vi "Filter_3Way.vi"(0 "Data IN":i32[](array[numeric]), 1 "DataRate (SPS)":dbl, 5 "Low Pass Filter Settings":T2, 7 "High Pass Filter Settings":T2, 9 "Notch Filter":enum16{"50Hz", "60Hz"}(ring)=enum."60Hz", 11 "Notch Order":i32, 12 "LPF Enable":bool, 13 "50/60 Notch Enable":bool, 14 "HPF Enable":bool) -> (4 "Data OUT":dbl[](array[numeric]))   [LabVIEW 2010]
doc: "This VI provides options for performing digitial filtering on the input data.\nOptions are provided for a single filter for each of the following:\n - Low Pass Filter\n - High Pass Filter\n - Notch Filter for 50/60Hz removal\n\nInputs;\nData IN - (I32[]) data to be filtered\nLPF Enable - (bool) TRUE = turn filter ON\nLow Pass Filter Settings - LPF parameters\nHPF Enable - (bool) TRUE = turn filter ON\nHigh Pass Filter Settings - HPF parameters\n50/60 Notch Enable - (bool) TRUE = turn filter ON\nNotch Filer - (enum) specify which filter to use\nNotch Order - (I32) notch filter order\nDataRate(SPS) - (DBL) data rate of input data\n\nOutput:\nData OUT - (DBL[]) filtered data"
uses:
  TYP_FilterSettings.ctl
  <vilib>/Analysis/3filter.llb/Filter Passband Type.ctl
  <vilib>/Analysis/3filter.llb/Butterworth Filter (DBL).vi
  <vilib>/Analysis/NI_AALBase.lvlib
panel:
  in  "50/60 Hz Notch Limits":T1={"50Hz Cutoff Freq"={"High"=53.0, "Low "=47.0}, "60Hz Cutoff Freq"={"High"=63.0, "Low "=57.0}} {"60Hz Cutoff Freq"."Low" format="%#_gHz"; "60Hz Cutoff Freq"."High" format="%#_gHz"; "50Hz Cutoff Freq"."Low" format="%#_gHz"; "50Hz Cutoff Freq"."High" format="%#_gHz"}
  # "Front Panel Constant (need to set as defaults)"
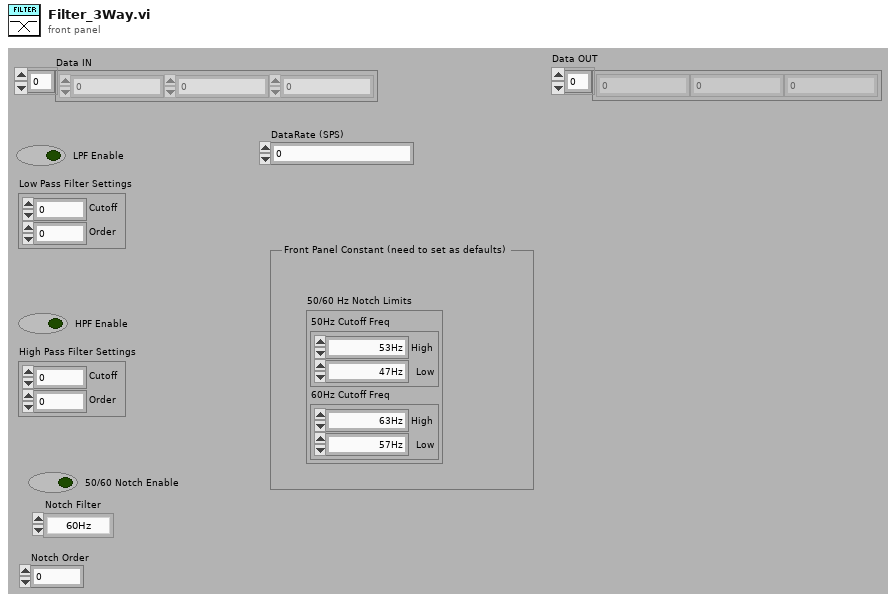
[diagram p1: front panel]
types:
  T1 = cluster{"50Hz Cutoff Freq":cluster{"High":dbl, "Low ":dbl}, "60Hz Cutoff Freq":cluster{"High":dbl, "Low ":dbl}}
  T2 = typedef "TYP_FilterSettings.ctl" = cluster{"Cutoff":dbl, "Order":i32}
  T3 = typedef "NI_AALBase.lvlib/Filter Passband Type.ctl" = enum32{"Lowpass", "Highpass", "Bandpass", "Bandstop"}
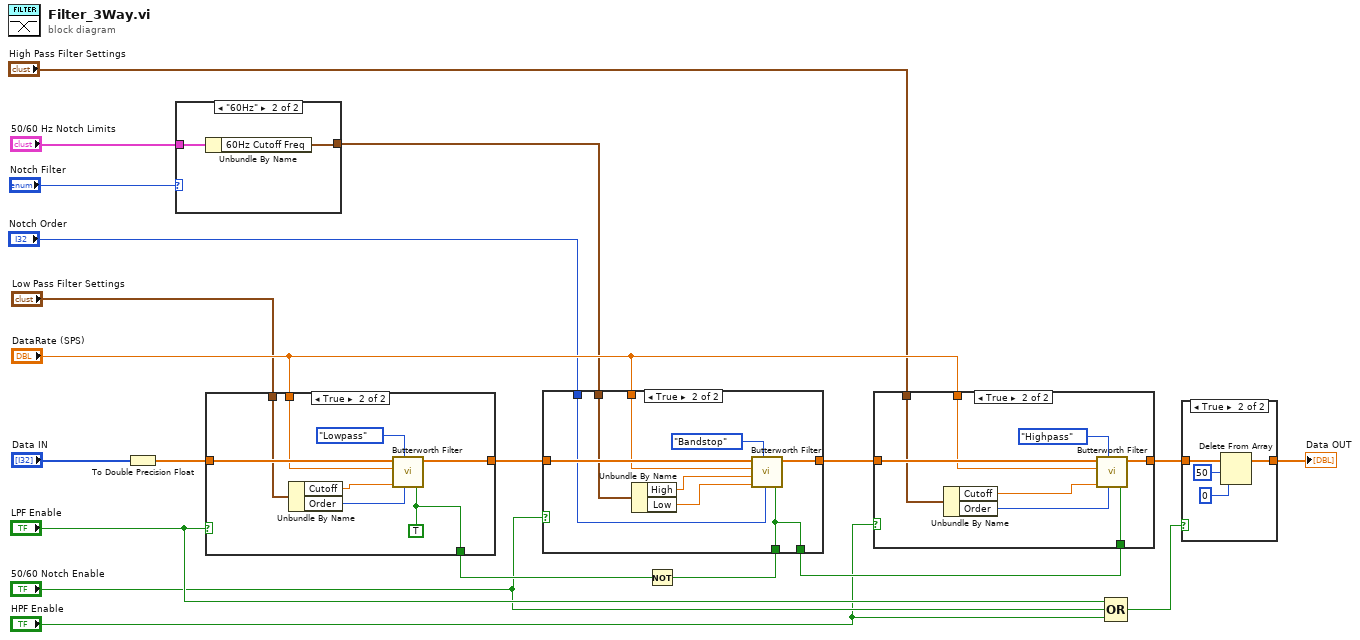
[diagram p0: block diagram]
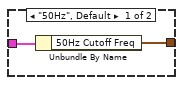
[diagram p3: hidden frame]
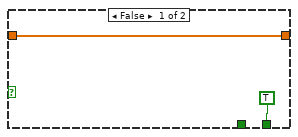
[diagram p5: hidden frame]
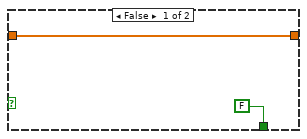
[diagram p6: hidden frame]
diagram:
  n1 = To Double Precision Float(number="Data IN") -> (double precision float=w17:dbl[])
  n2 = case shown="\"60Hz\"" "Notch Filter" {
    tunnel: "50/60 Hz Notch Limits" -> [w22 w24]
    tunnel: [w21 w23] -> w11
    frame "50Hz", Default {
      n3 = Unbundle By Name(w22) -> ("50Hz Cutoff Freq"=w21:cluster{"High":dbl, "Low ":dbl})
    }
    frame "60Hz" {
      n4 = Unbundle By Name(w24) -> ("60Hz Cutoff Freq"=w23:cluster{"High":dbl, "Low ":dbl})
    }
  }
  n5 = case shown="True" "LPF Enable" {
    tunnel: w17 -> [w26 w33]
    tunnel: [w26 w34] -> w19
    tunnel: "DataRate (SPS)" -> [_ w31]
    tunnel: "Low Pass Filter Settings" -> [_ w30]
    tunnel: [FALSE w27] -> w9
    frame False {
    }
    frame True {
      w27 = TRUE ("init/cont (init:F)")
      n6 = Unbundle By Name(w30) -> ("Cutoff"=w29:dbl, "Order"=w28:i32)
      n7 = call-poly <vilib>:"Butterworth Filter.vi"("init/cont (init:F)"=w27, "order"=w28, "filter type"=Filter_Passband_Type."Lowpass", "low cutoff freq: fl"=w29, "sampling freq: fs"=w31, "X"=w33) -> ("Filtered X"=w34:dbl[])  [unwired: 2 in, 1 out]
    }
  }
  n8 = Not(x=w9) -> (.not. x?=w8:bool)
  n9 = case shown="True" "50/60 Notch Enable" {
    tunnel: w19 -> [w36 w44]
    tunnel: [w36 w45] -> w18
    tunnel: "DataRate (SPS)" -> [_ w42]
    tunnel: "Notch Order" -> [_ w41]
    tunnel: w11 -> [_ w40]
    tunnel: w8 -> [_ w37]
    tunnel: [TRUE w37] -> w7
    frame False {
    }
    frame True {
      n10 = Unbundle By Name(w40) -> ("High"=w39:dbl, "Low"=w38:dbl)
      n11 = call-poly <vilib>:"Butterworth Filter.vi"("init/cont (init:F)"=w37, "order"=w41, "filter type"=Filter_Passband_Type."Bandstop", "low cutoff freq: fl"=w38, "high cutoff freq: fh"=w39, "sampling freq: fs"=w42, "X"=w44) -> ("Filtered X"=w45:dbl[])  [unwired: 1 in, 1 out]
    }
  }
  n12 = case shown="True" "HPF Enable" {
    tunnel: w18 -> [w46 w53]
    tunnel: [w46 w54] -> w6
    tunnel: "DataRate (SPS)" -> [_ w51]
    tunnel: "High Pass Filter Settings" -> [_ w50]
    tunnel: w7 -> [_ w47]
    frame False {
    }
    frame True {
      n13 = Unbundle By Name(w50) -> ("Cutoff"=w48:dbl, "Order"=w49:i32)
      n14 = call-poly <vilib>:"Butterworth Filter.vi"("init/cont (init:F)"=w47, "order"=w49, "filter type"=Filter_Passband_Type."Highpass", "low cutoff freq: fl"=w48, "sampling freq: fs"=w51, "X"=w53) -> ("Filtered X"=w54:dbl[])  [unwired: 2 in, 1 out]
    }
  }
  n15 = Compound Arithmetic op=OR("LPF Enable", "50/60 Notch Enable", "HPF Enable") -> (w1:bool)
  n16 = case shown="True" w1 {
    tunnel: w6 -> [w55 w59]
    tunnel: [w55 w58] -> w5
    frame False {
    }
    frame True {
      n17 = Delete From Array(array=w59, length=50, index=0) -> (array with subset deleted=w58:dbl[])  [unwired: 1 out]
    }
  }
  "Data OUT" <- w5
